vi "Cpx2Polar.vi"(5 "Real":dbl, 9 "Imag":dbl) -> (6 "Mag":dbl, 10 "Phase":dbl)   [LabVIEW 2014]
uses:
  <vilib>/Analysis/coordinate.llb/Angle Range (Degree).ctl
  <vilib>/Analysis/coordinate.llb/Angle Units.ctl
  <vilib>/Analysis/coordinate.llb/Wrap Angle (scalar).vi
  <vilib>/Analysis/NI_AAL_Angle.lvlib
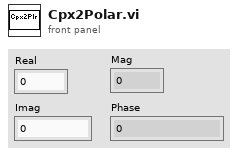
[diagram p1: front panel]
types:
  T1 = typedef "NI_AAL_Angle.lvlib/Angle Units.ctl" = i32
  T2 = typedef "NI_AAL_Angle.lvlib/Angle Range (Degree).ctl" = u16
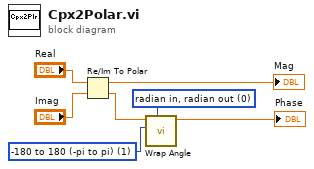
[diagram p0: block diagram]
diagram:
  w1 = T1 0 items=["radian in, radian out", "radian in, degree out", "degree in, degree out", "degree in, radian out"] ("angle units")
  w5 = T2 1 items=["none", "-180 to 180 (-pi to pi)", "0 to 360 (0 to 2pi)"] ("angle range")
  n1 = Re/Im To Polar(2:"Imag", 3:"Real") -> (0:w4:dbl, 1:→"Mag":dbl)
  n2 = call-poly <vilib>:"Wrap Angle.vi"("angle units"=w1, "angle range"=w5, "angle in"=w4) -> ("angle out"=→"Phase":dbl)  [unwired: 7 in, 1 out]
